vi "writeAccuracyFirgelli.vi"(8 "error in (no error)":errorcluster, 9 "maxLength":dbl=100.0, 10 "accuracy":dbl(slide)=100.0 scale=0.0..100.0 scale format="%.1f", 11 "handleIn":u32 format="%x") -> (0 "error out":errorcluster, 1 "regSetting":u16, 2 "pDataOut":u8[](array[numeric]), 3 "handleOut":u32 format="%x")   [LabVIEW 2019]
doc: "0x01 SET_ACCURACY:\nThis is the value controlled by the Accuracy Potentiometer. A value between 0-1023 is accepted. When the feedback position is plus or minus this value, the actuator will stop moving. Reducing this too far will result in the actuator continuously moving back and forth, never reaching the set point. The default value is four. To find the equivalent distance, use the formula:\n\nWritten by: Complete Automated Solutions\nwww.CompleteAutomatedSolutions.com"
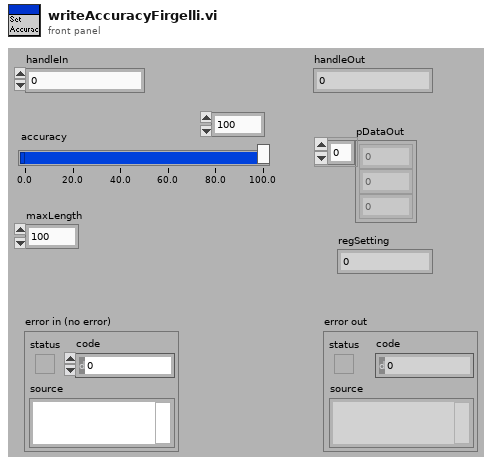
[diagram p1: front panel]
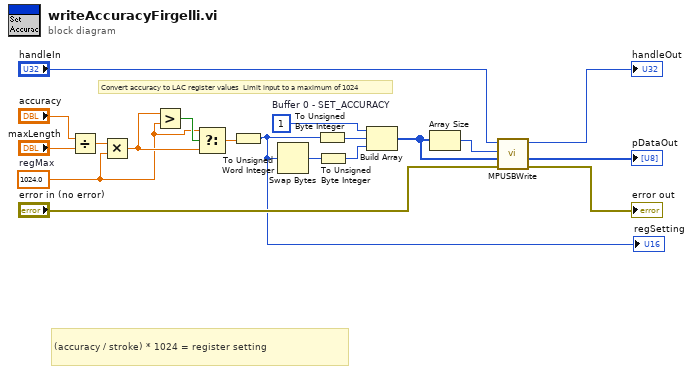
[diagram p0: block diagram]
diagram:
  w1 = 1024.0  # regMax
  w16 = u8 1  # Buffer 0 - SET_ACCURACY
  # "(accuracy / stroke) * 1024 = register setting"
  # "Convert accuracy to LAC register values  Limit input to a maximum of 1024"
  n1 = Divide(x="accuracy", y="maxLength") -> (x/y=w2:dbl)
  n2 = Multiply(x=w2, y=w1) -> (x*y=w5:dbl)
  n3 = Greater?(x=w5, y=w1) -> (0:w4:bool)
  n4 = Select(t=w1, s=w4, f=w5) -> (s? t:f=w6:dbl)
  n5 = To Unsigned Word Integer(number=w6) -> (unsigned 16bit integer=w9:u16)
  "regSetting" <- w9
  n6 = Swap Bytes(anything=w9) -> (byte swapped=w19:u16)
  n7 = To Unsigned Byte Integer(number=w9) -> (unsigned 8bit integer=w17:u8)
  n8 = To Unsigned Byte Integer(number=w19) -> (unsigned 8bit integer=w18:u8)
  n9 = Build Array(w16, w17, w18) -> (w14:u8[])
  n10 = Array Size(array=w14) -> (size(s)=w15:i32)
  n11 = call "MPUSBWrite.vi"("error in (no error)"="error in (no error)", "pDataIn"=w14, "dwLen"=w15, "handleIn"="handleIn") -> ("error out"=→"error out":errorcluster, "pDataOut"=→"pDataOut":u8[], "handleOut"=→"handleOut":u32)  [unwired: 2 in, 3 out]
